vi "color changing using property node.vi"() -> ()   [LabVIEW 2018]
panel:
  out "Slide":u8(slide) scale=0.0..100.0
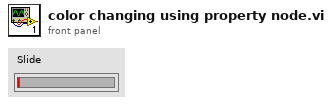
[diagram p1: front panel]
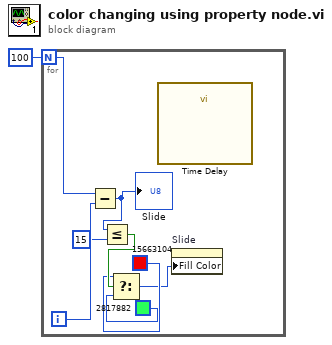
[diagram p0: block diagram]
diagram:
  n1 = for {
    N: 100 -> [w8]
    i -> [w9]
    n2 = Subtract(x=w8, y=w9) -> (x-y=w7:i32)
    "Slide" <- w7
    n3 = Less Or Equal?(x=w7, y=15) -> (x <= y?=w5:bool)
    n4 = Select(t=u32 15663104, s=w5, f=u32 2817882) -> (s? t:f=w2:u32)
    n5 = call "Time Delay"() -> ()  [unwired: 11 in, 1 out]
    n6 = property on="Slide" class="Slide (strict)"("Fill Color"=w2) -> ()  [unwired: 2 in, 2 out]
  }
